vi "no_standing_test6_R.vi"(4 "t_ext_default":i32, 6 "t_flex_default":i32, 7 "Reset zero":bool, 8 "peak ratio":dbl, 9 "extension ratio":dbl, 10 "flexion ratio":dbl, 11 "Hip angle":dbl(knob) scale=-20.0..50.0) -> (0 "Extension torque":dbl, 3 "Flexion torque":dbl)   [LabVIEW 2019]
uses:
  <vilib>/functionblocks/Edge Detection/One Shot Rising with Input/One Shot Rising with Input.vi
  <vilib>/functionblocks/FB Core/FB Core.xnode
  <vilib>/functionblocks/NI_FunctionBlock Libraries.lvlib
panel:
  out "output1 (int) 2":dbl
  out "output1 (int)":dbl
  out "a_ext":dbl
  out "x_ext_val":i32
  out "x_ext":i32
  out "a_flex":dbl
  out "x_flex_val":i32
  out "x_flex":i32
  out "standing":bool
  out "extension phase":u32
  out "flexion phase":u32
  out "ext eq":dbl
  out "flex eq":dbl
  out "Flexion":bool
  out "Ext Eq.":dbl
  out "Flex Eq.":dbl
  out "ROM":dbl
  out "min":dbl
  out "max":dbl
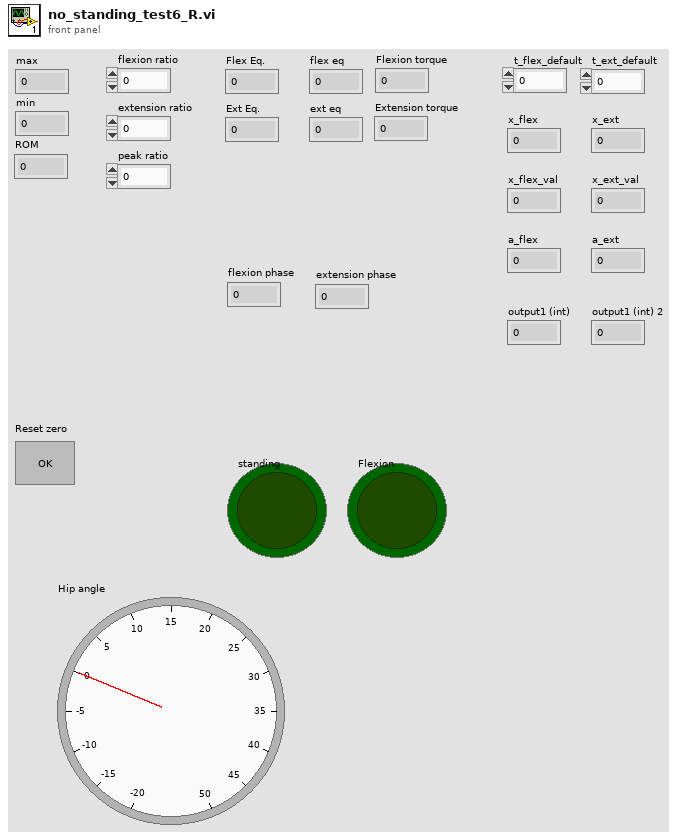
[diagram p1: front panel]
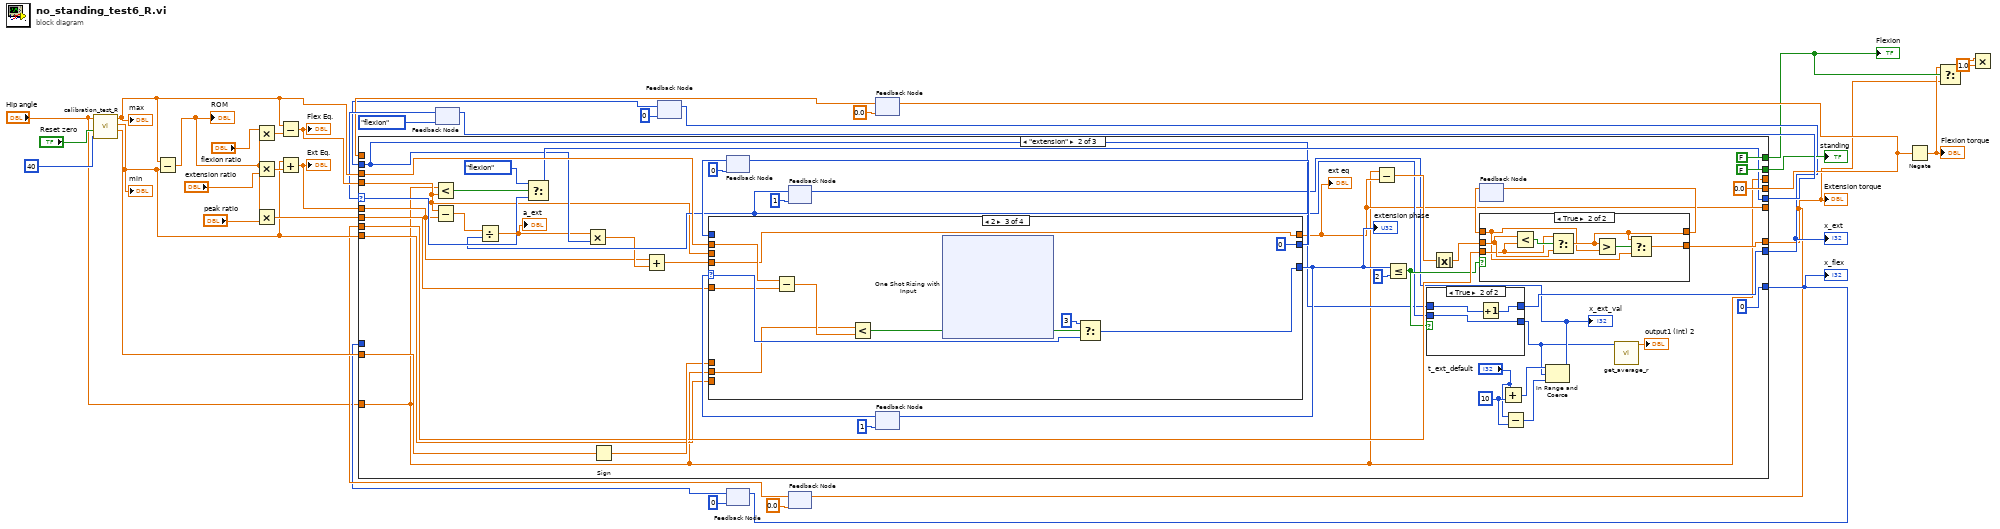
[diagram p0: block diagram]
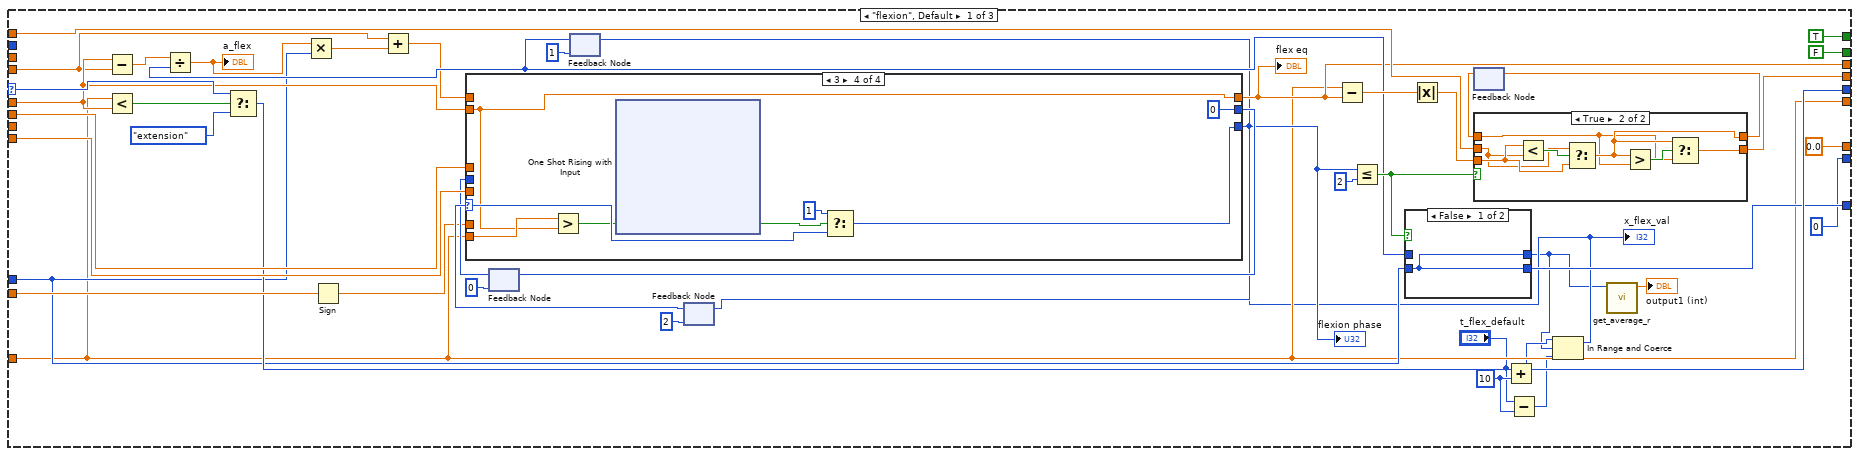
[diagram p2: hidden frame]
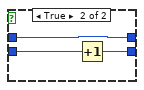
[diagram p3: hidden frame]
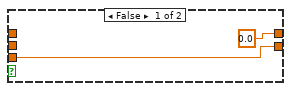
[diagram p4: hidden frame]
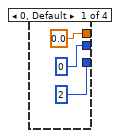
[diagram p5: hidden frame]
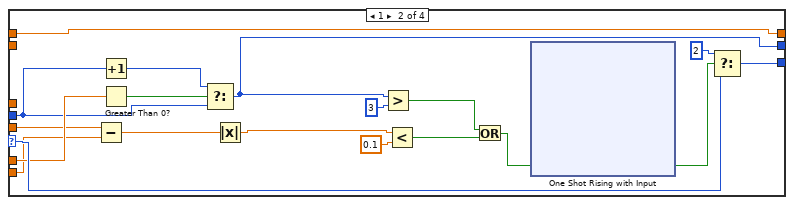
[diagram p6: hidden frame]
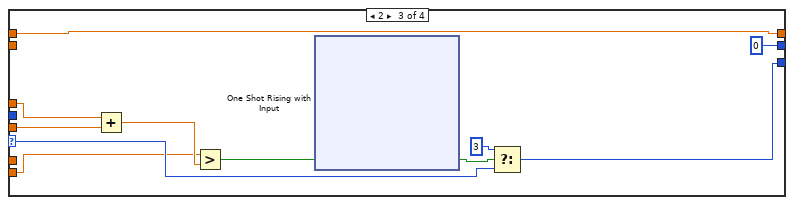
[diagram p7: hidden frame]
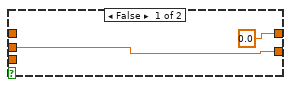
[diagram p9: hidden frame]
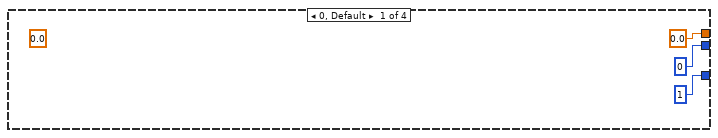
[diagram p10: hidden frame]
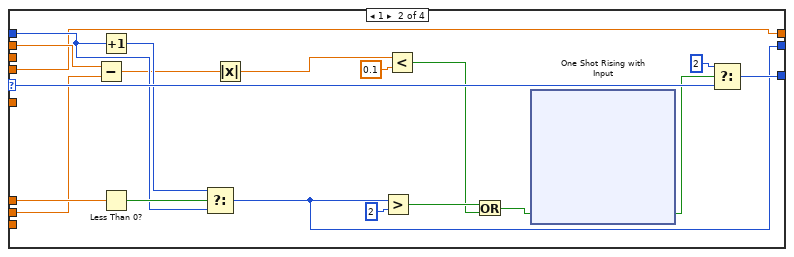
[diagram p11: hidden frame]
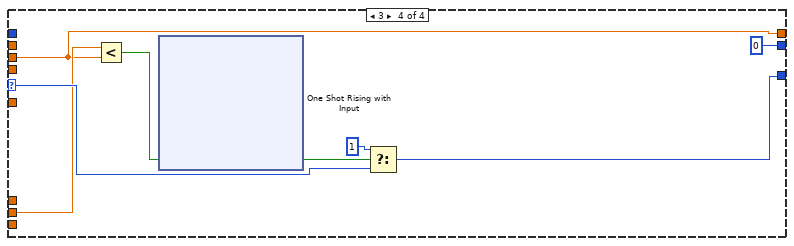
[diagram p12: hidden frame]
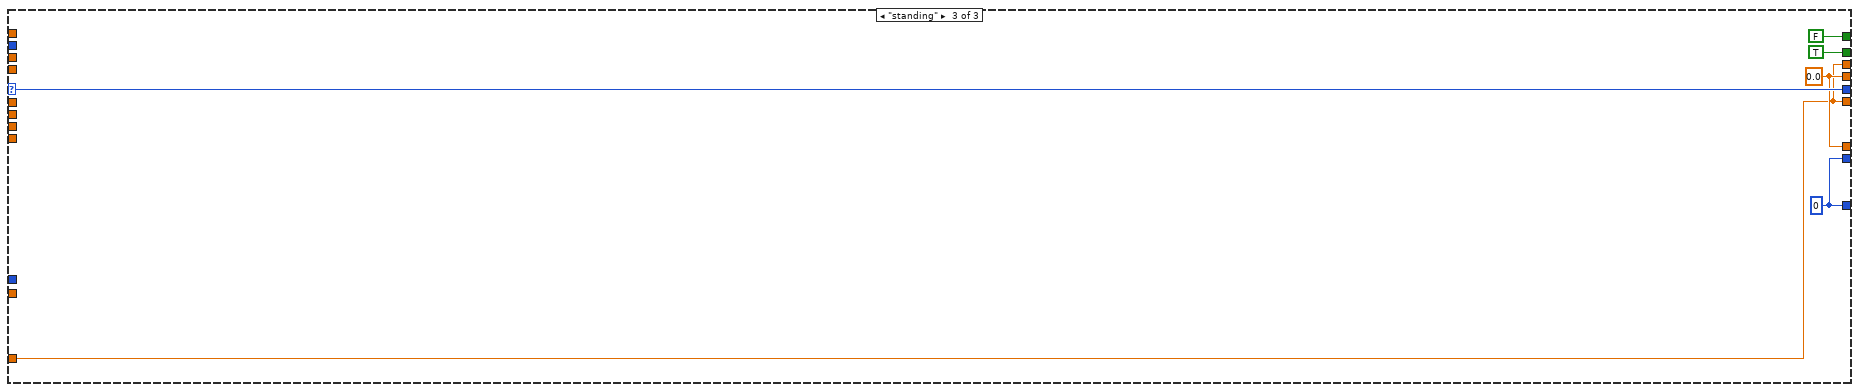
[diagram p13: hidden frame]
diagram:
  n1 = call "calibration_test_R.vi"("i_pos_thres"=40 ("ext peak thres"), "Reset zero"="Reset zero", "Hip angle"="Hip angle") -> ("diff"=w21:dbl, "min"=w24:dbl, "max"=w25:dbl)  [unwired: 4 in, 1 out]
  "max" <- w25
  "min" <- w24
  n2 = Subtract(x=w25, y=w24) -> (x-y=w3:dbl)
  "ROM" <- w3
  n3 = Multiply(x="flexion ratio", y=w3) -> (x*y=w34:dbl)
  n4 = Multiply(x=w3, y="extension ratio") -> (x*y=w28:dbl)
  n5 = Multiply(x=w3, y="peak ratio") -> (x*y=w31:dbl)
  n6 = Subtract(x=w25, y=w34) -> (x-y=w33:dbl)
  "Flex Eq." <- w33
  n7 = Add(x=w24, y=w28) -> (x+y=w30:dbl)
  "Ext Eq." <- w30
  n8 = feedback #1(enum16{"flexion", "extension", "standing"}."flexion") -> (w22:enum16{"flexion", "extension", "standing"})
  n9 = feedback #2(0) -> (w10:i32)
  n10 = feedback #3(0) -> (w14:i32)
  n11 = feedback #4(0.0 ("Ext Eq.")) -> (w15:dbl)
  n12 = feedback #5(0.0 ("Ext Eq.")) -> (w19:dbl)
  n13 = case shown="\"extension\"" w22 {
    selector: w22 -> [w67 w280 w467]
    tunnel: [w69 w281 w467] -> w29
    tunnel: "Hip angle" -> [w43 w256 w463]
    tunnel: w33 -> [w47 w260 _]
    tunnel: w30 -> [w53 w258 _]
    tunnel: [w59 0.0 ("Ext Eq.") w466] -> w17
    tunnel: w24 -> [w80 w262 _]
    tunnel: w31 -> [w79 w289 _]
    tunnel: [0.0 w273 w466] -> w6
    tunnel: w25 -> [_ w290 _]
    tunnel: w21 -> [w70 w282 _]
    tunnel: [TRUE FALSE FALSE] -> w8
    tunnel: [FALSE FALSE TRUE] -> w20
    tunnel: w19 -> [w62 _ _]
    tunnel: w15 -> [_ w272 _]
    tunnel: w14 -> [w49 _ _]
    tunnel: [w55 0 w464] -> w13
    tunnel: w10 -> [_ w265 _]
    tunnel: [0 w269 w464] -> w9
    tunnel: [w43 w257 w463] -> _
    tunnel: [w44 w256 w463] -> _
    frame "flexion", Default {
      w41 = 10 ("y")
      n14 = Subtract(x=w53, y=w47) -> (x-y=w52:dbl)
      n15 = Less?(x=w43, y=w53) -> (x < y?=w68:bool)
      n16 = Select(t=w67, s=w68, f=enum16{"flexion", "extension", "standing"}."extension") -> (s? t:f=w69:enum16{"flexion", "extension", "standing"})
      n17 = Sign(1:w70) -> (0:w71:dbl)
      n18 = feedback #6(0) -> (w74:i32)
      n19 = feedback #7(1) -> (w51:i32)
      n20 = Divide(x=w52, y=w51) -> (x/y=w50:dbl)
      "a_flex" <- w50
      n21 = Multiply(x=w50, y=w49) -> (x*y=w48:dbl)
      n22 = Add(x=w47, y=w48) -> (x+y=w46:dbl)
      n23 = feedback #8(u32 2 ("milliseconds to wait")) -> (w76:u32)
      n24 = case shown="3" w76 {
        selector: w76 -> [_ w113 w162 w208]
        tunnel: [0.0 w97 w154 w206] -> w44
        tunnel: w53 -> [_ _ _ w206]
        tunnel: w80 -> [_ w103 w161 _]
        tunnel: w43 -> [_ w102 w158 w207]
        tunnel: [u32 2 ("milliseconds to wait") w115 w163 w209] -> w58
        tunnel: w79 -> [_ _ w160 _]
        tunnel: w71 -> [_ w112 _ _]
        tunnel: [0 w108 0 0] -> w75
        tunnel: w74 -> [_ w109 _ _]
        tunnel: w46 -> [_ w97 w154 _]
        frame 0, Default {
        }
        frame 1 {
          n25 = Subtract(x=w103, y=w102) -> (x-y=w106:dbl)
          n26 = Increment(x=w109) -> (x+1=w110:i32)
          n27 = Greater Than 0?(x=w112) -> (x > 0?=w111:bool)
          n28 = Select(t=w110, s=w111, f=w109) -> (s? t:f=w108:i32)
          n29 = Absolute Value(x=w106) -> (abs(x)=w105:dbl)
          n30 = Greater?(x=w108, y=3) -> (0:w101:bool)
          n31 = Less?(x=w105, y=0.1) -> (x < y?=w100:bool)
          n32 = Or(x=w101, y=w100) -> (x .or. y?=w99:bool)
          n33 = xnode "One Shot Rising with Input"("input"=w99) -> ("output"=w98:bool)  [unwired: 1 in, 1 out]
          n34 = Select(t=u32 2 ("milliseconds to wait"), s=w98, f=w113) -> (s? t:f=w115:u32)
        }
        frame 2 {
          n35 = Add(x=w160, y=w161) -> (x+y=w159:dbl)
          n36 = Greater?(x=w158, y=w159) -> (0:w156:bool)
          n37 = xnode "One Shot Rising with Input"("input"=w156) -> ("output"=w155:bool)  [unwired: 1 in, 1 out]
          n38 = Select(t=u32 3 ("milliseconds to wait"), s=w155, f=w162) -> (s? t:f=w163:u32)
        }
        frame 3 {
          n39 = Greater?(x=w207, y=w206) -> (0:w204:bool)
          n40 = xnode "One Shot Rising with Input"("input"=w204) -> ("output"=w203:bool)  [unwired: 1 in, 1 out]
          n41 = Select(t=u32 1 ("milliseconds to wait"), s=w203, f=w208) -> (s? t:f=w209:u32)
        }
      }
      "flex eq" <- w44
      "flexion phase" <- w58
      n42 = feedback-in #6(w75) -> ()
      n43 = feedback-in #8(w58) -> ()
      n44 = Subtract(x=w43, y=w44) -> (x-y=w63:dbl)
      n45 = Less Or Equal?(x=w58, y=u32 2) -> (x <= y?=w56:bool)
      n46 = case shown="False" w56 {
        tunnel: [w81 w84] -> w55
        tunnel: w49 -> [w81 w83]
        tunnel: [w81 w82] -> w36
        tunnel: w51 -> [_ w82]
        frame False {
        }
        frame True {
          n47 = Increment(x=w83) -> (x+1=w84:i32)
        }
      }
      n48 = Absolute Value(x=w63) -> (abs(x)=w57:dbl)
      n49 = feedback #9() -> (w60:dbl)  [unwired: 1 in]
      n50 = case shown="True" w56 {
        tunnel: w62 -> [_ w91]
        tunnel: w57 -> [w86 w92]
        tunnel: [0.0 ("Ext Eq.") w88] -> w61
        tunnel: w60 -> [_ w87]
        tunnel: [w86 w89] -> w59
        frame False {
        }
        frame True {
          n51 = Less?(x=w92, y=w91) -> (x < y?=w93:bool)
          n52 = Select(t=w91, s=w93, f=w92) -> (s? t:f=w88:dbl)
          n53 = Greater?(x=w88, y=w87) -> (0:w90:bool)
          n54 = Select(t=w88, s=w90, f=w87) -> (s? t:f=w89:dbl)
        }
      }
      n55 = feedback-in #9(w61) -> ()
      n56 = Add(x="t_flex_default", y=w41) -> (x+y=w39:i32)
      n57 = Subtract(x="t_flex_default", y=w41) -> (x-y=w40:i32)
      n58 = In Range and Coerce(upper limit=w39, x=w36, lower limit=w40) -> (coerced(x)=w37:i32)  [unwired: 1 out]
      "x_flex_val" <- w37
      n59 = feedback-in #7(w37) -> ()
      n60 = call "get_average_r.vi"("input1 (int)"=w36) -> ("output1 (int)"=→"output1 (int)":dbl)  [unwired: 9 in, 1 out]
    }
    frame "extension" {
      w253 = 10 ("y")
      n61 = Less?(x=w256, y=w260) -> (x < y?=w279:bool)
      n62 = Subtract(x=w260, y=w258) -> (x-y=w264:dbl)
      n63 = Select(t=enum16{"flexion", "extension", "standing"}."flexion", s=w279, f=w280) -> (s? t:f=w281:enum16{"flexion", "extension", "standing"})
      n64 = Sign(1:w282) -> (0:w284:dbl)
      n65 = feedback #10(0) -> (w287:i32)
      n66 = feedback #11(1) -> (w266:i32)
      n67 = Divide(x=w264, y=w266) -> (x/y=w259:dbl)
      "a_ext" <- w259
      n68 = Multiply(x=w259, y=w265) -> (x*y=w263:dbl)
      n69 = Add(x=w258, y=w263) -> (x+y=w261:dbl)
      n70 = feedback #12(u32 1 ("milliseconds to wait")) -> (w293:u32)
      n71 = case shown="2" w293 {
        selector: w293 -> [_ w329 w378 w423]
        tunnel: [u32 1 ("milliseconds to wait") w327 w377 w424] -> w276
        tunnel: [0.0 w311 w368 w420] -> w257
        tunnel: w260 -> [_ _ _ w420]
        tunnel: w290 -> [_ w321 w375 _]
        tunnel: w256 -> [_ w318 w372 w421]
        tunnel: w289 -> [_ _ w374 _]
        tunnel: w284 -> [_ w324 _ _]
        tunnel: [0 w317 0 0] -> w286
        tunnel: w287 -> [_ w323 _ _]
        tunnel: w262 -> [_ _ _ _]
        tunnel: w261 -> [_ w311 w368 _]
        frame 0, Default {
          (unwired) 0.0
        }
        frame 1 {
          n72 = Subtract(x=w321, y=w318) -> (x-y=w322:dbl)
          n73 = Increment(x=w323) -> (x+1=w325:i32)
          n74 = Less Than 0?(x=w324) -> (x < 0?=w326:bool)
          n75 = Select(t=w325, s=w326, f=w323) -> (s? t:f=w317:i32)
          n76 = Absolute Value(x=w322) -> (abs(x)=w320:dbl)
          n77 = Greater?(x=w317, y=2) -> (0:w315:bool)
          n78 = Less?(x=w320, y=0.1) -> (x < y?=w314:bool)
          n79 = Or(x=w315, y=w314) -> (x .or. y?=w313:bool)
          n80 = xnode "One Shot Rising with Input"("input"=w313) -> ("output"=w312:bool)  [unwired: 1 in, 1 out]
          n81 = Select(t=u32 2, s=w312, f=w329) -> (s? t:f=w327:u32)
        }
        frame 2 {
          n82 = Subtract(x=w375, y=w374) -> (x-y=w373:dbl)
          n83 = Less?(x=w372, y=w373) -> (x < y?=w370:bool)
          n84 = xnode "One Shot Rising with Input"("input"=w370) -> ("output"=w369:bool)  [unwired: 1 in, 1 out]
          n85 = Select(t=u32 3, s=w369, f=w378) -> (s? t:f=w377:u32)
        }
        frame 3 {
          n86 = Less?(x=w421, y=w420) -> (x < y?=w418:bool)
          n87 = xnode "One Shot Rising with Input"("input"=w418) -> ("output"=w417:bool)  [unwired: 1 in, 1 out]
          n88 = Select(t=u32 1, s=w417, f=w423) -> (s? t:f=w424:u32)
        }
      }
      "ext eq" <- w257
      "extension phase" <- w276
      n89 = feedback-in #10(w286) -> ()
      n90 = feedback-in #12(w276) -> ()
      n91 = Subtract(x=w256, y=w257) -> (x-y=w291:dbl)
      n92 = Less Or Equal?(x=w276, y=u32 2) -> (x <= y?=w267:bool)
      n93 = case shown="True" w267 {
        tunnel: [w295 w298] -> w269
        tunnel: w265 -> [w295 w297]
        tunnel: [w295 w296] -> w249
        tunnel: w266 -> [_ w296]
        frame False {
        }
        frame True {
          n94 = Increment(x=w297) -> (x+1=w298:i32)
        }
      }
      n95 = Absolute Value(x=w291) -> (abs(x)=w274:dbl)
      n96 = feedback #13() -> (w277:dbl)  [unwired: 1 in]
      n97 = case shown="True" w267 {
        tunnel: w272 -> [_ w305]
        tunnel: w274 -> [w300 w306]
        tunnel: [0.0 ("Ext Eq.") w302] -> w271
        tunnel: w277 -> [_ w301]
        tunnel: [w300 w303] -> w273
        frame False {
        }
        frame True {
          n98 = Less?(x=w306, y=w305) -> (x < y?=w307:bool)
          n99 = Select(t=w305, s=w307, f=w306) -> (s? t:f=w302:dbl)
          n100 = Greater?(x=w302, y=w301) -> (0:w304:bool)
          n101 = Select(t=w302, s=w304, f=w301) -> (s? t:f=w303:dbl)
        }
      }
      n102 = feedback-in #13(w271) -> ()
      n103 = Add(x="t_ext_default", y=w253) -> (x+y=w254:i32)
      n104 = Subtract(x="t_ext_default", y=w253) -> (x-y=w252:i32)
      n105 = In Range and Coerce(upper limit=w254, x=w249, lower limit=w252) -> (coerced(x)=w250:i32)  [unwired: 1 out]
      "x_ext_val" <- w250
      n106 = feedback-in #11(w250) -> ()
      n107 = call "get_average_r.vi"("input1 (int)"=w249) -> ("output1 (int)"=→"output1 (int) 2":dbl)  [unwired: 9 in, 1 out]
    }
    frame "standing" {
      w464 = 0
      w466 = 0.0
    }
  }
  "Flexion" <- w8
  "Extension torque" <- w6
  "standing" <- w20
  "x_flex" <- w13
  "x_ext" <- w9
  n108 = feedback-in #1(w29) -> ()
  n109 = feedback-in #2(w9) -> ()
  n110 = feedback-in #3(w13) -> ()
  n111 = feedback-in #4(w6) -> ()
  n112 = feedback-in #5(w17) -> ()
  n113 = Negate(x=w17) -> (-x=w7:dbl)
  "Flexion torque" <- w7
  n114 = Select(t=w7, s=w8, f=w6) -> (s? t:f=w4:dbl)
  n115 = Multiply(x=w4, y=1.0) -> ()  [unwired: 1 out]
